vi "Update Taps.vi"(6 "Gradient":i16, 9 "Taps":refnum<k21>, 11 "Weights":refnum<k21>) -> (1 "Taps Out":refnum<k21>, 3 "Weights Out":refnum<k21>, 5 "FIR Out":fxp<+/-,32,24> format="%.31g")   [LabVIEW 2017]
uses:
  <vilib>/rvi/Emulation/niFpgaSctlEmulationGetInTimedLoop.vi
  <vilib>/Utility/error.llb/Clear Errors.vi
  <vilib>/rvi/DataTransferAndStorage/Container/Common/niFpgaContainerExecOnDevCompGetState.vi
  <vilib>/rvi/Emulation/niFpgaEmulationIsFPGAContextNoSignature.vi
  <vilib>/rvi/DataTransferAndStorage/Container/Common/niFpgaContainerGetUniqueNameForEmu.vi
  <vilib>/rvi/Emulation/niFpgaProcessEmulError.vi
  <vilib>/rvi/errors/nirviReportUnexpectedCaseInternalError (U32).vi
  <vilib>/rvi/Memory/Memory_Emulation/niFpgaMemoryEmulationCacheClearOnFirstRun.vi
  <vilib>/rvi/Memory/Memory_Emulation/nirvimemoryEmulationManagerCache_MakeExclusive.vi
  <vilib>/rvi/Memory/Memory_Emulation/niFpgaMemoryEmulationValidateCache.vi
  <vilib>/rvi/Memory/Memory_Emulation/nirvimemoryEmulationManagerCache_InsertValue.vi
  <vilib>/rvi/Memory/Memory_Emulation/nirvimemoryEmulationManagerCache_ReleaseExclusive.vi
  <vilib>/rvi/Memory/Memory_Emulation/nirvimemoryEmulationManagerCache_GetValue.vi
  <vilib>/rvi/Memory/Memory_Emulation/nirvimemoryEmulationManagerCache_SetValue.vi
  <vilib>/rvi/Emulation/niFpgaSctlEmulationResourceMgr.vi
  <vilib>/rvi/DataTransferAndStorage/Container/XNode/niFpgaContainer.xnode
  <vilib>/rvi/Memory/Memory_Emulation/niFpgaMemoryEmulationRefIn.vi
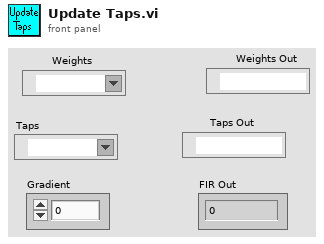
[diagram p1: front panel]
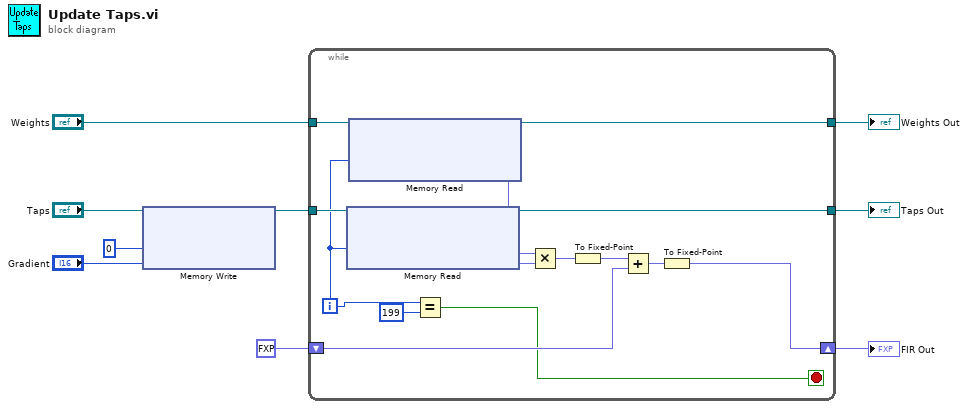
[diagram p0: block diagram]
diagram:
  n1 = xnode ("Memory Write")("Address"=u32 0, "Data"="Gradient", "Memory In"="Taps") -> ("Memory Out"=w7:refnum<k21>)
  n2 = while {
    tunnel: "Weights" -> [w23]
    tunnel: w7 -> [w22]
    shift-right: [w13] -> w4
    shift-left: fxp<+/-,32,24> 0.0 ("x+y") -> [w14]
    tunnel: [w17] -> w3
    tunnel: [w16] -> w2
    i -> [w12]
    stop <- w10 stop-if-true
    n3 = xnode ("Memory Read")("Address"=w12, "Memory In"=w22) -> ("Data"=w20:fxp<+/-,32,24>, "Memory Out"=w16:refnum<k21>)
    n4 = xnode ("Memory Read")("Address"=w12, "Memory In"=w23) -> ("Data"=w21:fxp<+/-,32,24>, "Memory Out"=w17:refnum<k21>)
    n5 = Equal?(x=w12, y=199) -> (x = y?=w10:bool)
    n6 = Multiply(x=w21, y=w20) -> (x*y=w19:fxp<+/-,64,48>)
    n7 = To Fixed-Point(number=w19) -> (fixed-point=w15:fxp<+/-,32,24>)  [unwired: 1 in]
    n8 = Add(x=w15, y=w14) -> (x+y=w18:fxp<+/-,33,25>)
    n9 = To Fixed-Point(number=w18) -> (fixed-point=w13:fxp<+/-,32,24>)  [unwired: 1 in]
  }
  "FIR Out" <- w4
  "Weights Out" <- w3
  "Taps Out" <- w2
